vi "Open Session.vi"(9 "Channels":enum16{"0", "1", "0,1"}(ring), 11 "x4xx argument":string="192.167.11.2") -> (0 "error out":errorcluster, 3 "Session Out":T1)   [LabVIEW 2023]
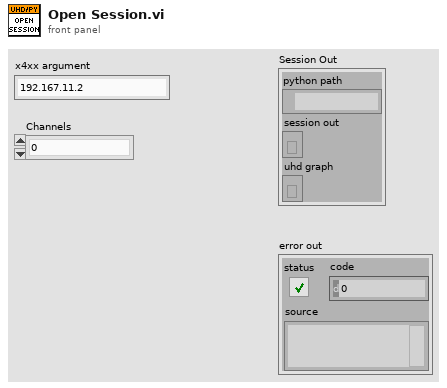
[diagram p1: front panel]
types:
  T1 = cluster{"python path":path, "session out":refnum<k35>, "uhd graph":refnum<k38>}
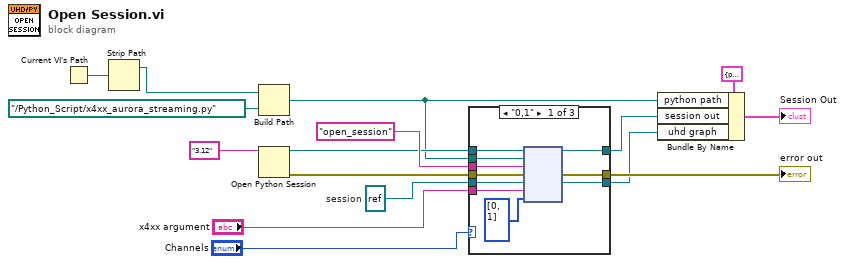
[diagram p0: block diagram]
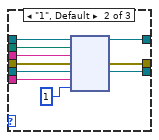
[diagram p2: hidden frame]
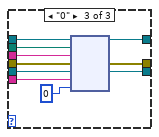
[diagram p3: hidden frame]
diagram:
  w10 = refnum<k38> refnum  # session
  n1 = Current VI's Path() -> (path=w14:path)
  n2 = Strip Path(path=w14) -> (stripped path=w15:path)  [unwired: 1 out]
  n3 = Build Path(base path=w15, name or relative path=path "../Python_Script/x4xx_aurora_streaming.py" ("module path")) -> (appended path=w6:path)
  n4 = Open Python Session(python version="3.12" ("Python version")) -> (session out=w8:refnum<k35>, error out=w12:errorcluster)  [unwired: 2 in]
  n5 = case shown="\"0,1\"" "Channels" {
    tunnel: w12 -> [w22 w36 w46]
    tunnel: [w21 w35 w45] -> w11
    tunnel: w10 -> [w20 w34 w44]
    tunnel: "open_session" ("function name") -> [w24 w33 w43]
    tunnel: w8 -> [w26 w32 w42]
    tunnel: w6 -> [w23 w31 w41]
    tunnel: [w25 w30 w40] -> w5
    tunnel: [w19 w29 w39] -> w4
    tunnel: "x4xx argument" -> [w18 w28 w38]
    frame "0,1" {
      n6 = node(w26, w23, w24, w22, w20, w18, i32[] [0, 1]) -> (w25:refnum<k35>, w21:errorcluster, w19:refnum<k38>)  [unwired: 2 in, 2 out]
    }
    frame "1", Default {
      n7 = node(w32, w31, w33, w36, w34, w28, 1) -> (w30:refnum<k35>, w35:errorcluster, w29:refnum<k38>)  [unwired: 2 in, 2 out]
    }
    frame "0" {
      n8 = node(w42, w41, w43, w46, w44, w38, 0) -> (w40:refnum<k35>, w45:errorcluster, w39:refnum<k38>)  [unwired: 2 in, 2 out]
    }
  }
  "error out" <- w11
  n9 = Bundle By Name(cluster=T1 {"python path"=path "", "session out"=refnum, "uhd graph"=refnum}, "python path"=w6, "session out"=w5, "uhd graph"=w4) -> (→"Session Out":T1)
